vi "Kinda Edge Detect Line.vi"() -> ()   [LabVIEW 2018]
uses:
  <vilib>/vision/driver/IMAQdx.llb/IMAQdx Camera Control Mode.ctl
  <vilib>/userdefined/High Color/IMAQdx.ctl
  <vilib>/vision/driver/NI_Vision_Acquisition_Software.lvlib
  <resource>/objmgr/imaqdx.rc
panel:
  out "element 2":T1
  out "Image Out 2":T2(plugin-control)
  in  "error in 3":errorcluster
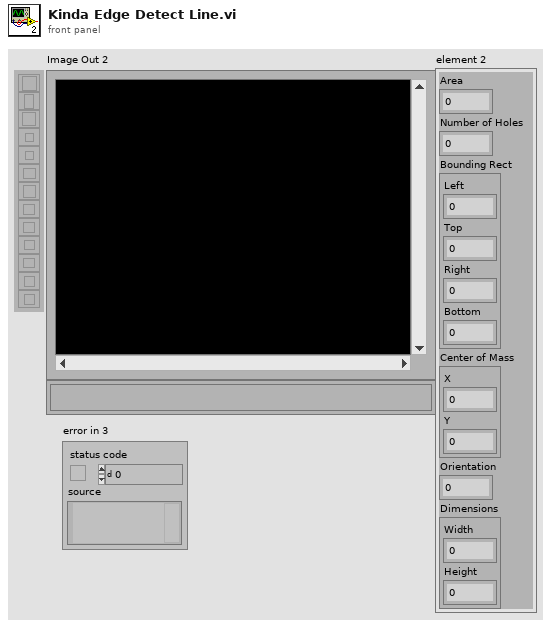
[diagram p1: front panel]
types:
  T1 = cluster{"Area":dbl, "Number of Holes":dbl, "Bounding Rect":cluster{"Left":dbl, "Top":dbl, "Right":dbl, "Bottom":dbl}, "Center of Mass":cluster{"X":dbl, "Y":dbl}, "Orientation":dbl, "Dimensions":cluster{"Width":dbl, "Height":dbl}}
  T2 = typedef "IMAQ Image.ctl" = refnum<image>
  T3 = typedef "IMAQdx.ctl" = refnum<k21>
  T4 = typedef "NI_Vision_Acquisition_Software.lvlib/IMAQdx Camera Control Mode.ctl" = enum32{"Controller", "Listener"}
  T5 = typedef "Image Type" = u32
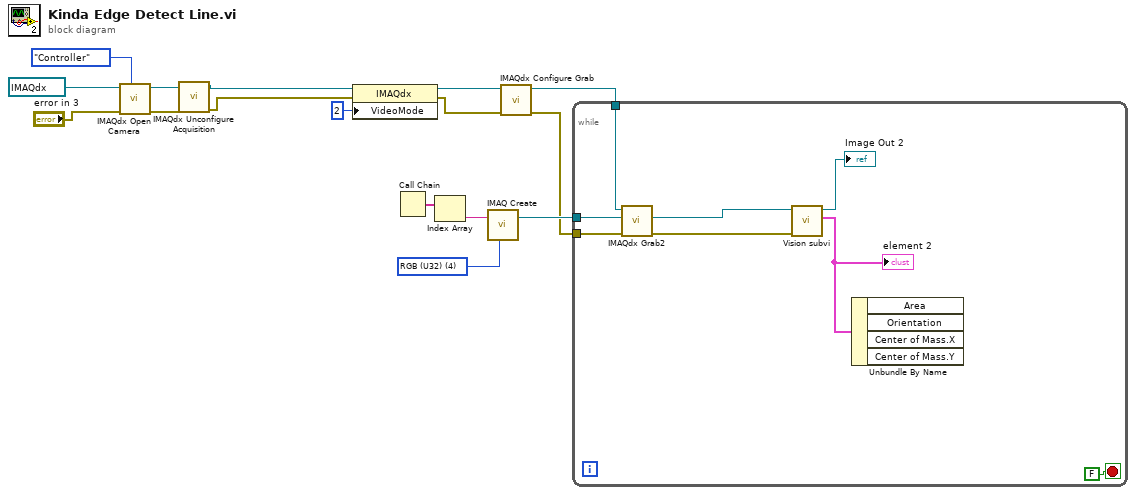
[diagram p0: block diagram]
diagram:
  w5 = T5 4 items=["Grayscale (U8)", "Grayscale (I16)", "Grayscale (SGL)", "Complex (CSG)", "RGB (U32)", "HSL (U32)", "RGB (U64)", "Grayscale (U16)"] ("Image Type")
  n1 = call <vilib>:"IMAQdx Open Camera.vi"("Camera Control Mode"=IMAQdx_Camera_Control_Mode."Controller", "error in"="error in 3", "Session In"=T3 "cam1") -> ("error out"=w10:errorcluster, "Session Out"=w11:T3)  [unwired: 7 in]
  n2 = call <vilib>:"IMAQdx Unconfigure Acquisition.vi"("error in"=w10, "Session In"=w11) -> ("error out"=w13:errorcluster, "Session Out"=w12:T3)  [unwired: 8 in]
  n3 = property class="IMAQdx"(reference=w12, error in=w13, "VideoMode"=u32 2) -> (reference out=w9:T3, error out=w1:errorcluster)
  n4 = Call Chain() -> (call chain=w7:string[])
  n5 = Index Array(array=w7) -> (element=w6:string)  [unwired: 1 in]
  n6 = call "IMAQ Create"("Image Name"=w6, "Image Type"=w5) -> ("New Image"=w15:T2)  [unwired: 2 in, 2 out]
  n7 = call <vilib>:"IMAQdx Configure Grab.vi"("error in"=w1, "Session In"=w9) -> ("error out"=w14:errorcluster, "Session Out"=w16:T3)  [unwired: 8 in]
  n8 = while {
    tunnel: w16 -> [w24]
    tunnel: w15 -> [w23]
    tunnel: w14 -> [w20]
    stop <- FALSE ("stop") stop-if-true
    n9 = call <vilib>:"IMAQdx Grab2.vi"("error in"=w20, "Image In"=w23, "Session In"=w24) -> ("error out"=w19:errorcluster, "Image Out"=w17:T2)  [unwired: 5 in, 2 out]
    n10 = call "Vision subvi.vi"("error in (no error)"=w19, "Image Src"=w17) -> ("element 2"=w18:T1, "Image Out 2"=→"Image Out 2":T2)  [unwired: 7 in, 1 out]
    "element 2" <- w18
    n11 = Unbundle By Name(w18) -> ()  [unwired: 4 out]
  }
